vi "Configure Flow Rate.vi"(5 "Retry Attempts (0)":i32 min=0, 8 "error in":errorcluster, 10 "Flow Input (ml/min)":dbl, 11 "VISA resource name":refnum<visa-resource-name>) -> (0 "error out":errorcluster, 3 "VISA resource name out":refnum<visa-resource-name>)   [LabVIEW 2020, in "ChromTech Series III Pump.lvlib"]
doc: "Configures the flow rate using up to 5 digits. If the entered value exceeds the maximum allowable flow rate of the pump, the flow rate will be automatically set to the maximum allowable flow rate. The maximum allowable flow rate can be found using the Get Maximum Flow Rate VI and the current flow rate can be found using the Get Current Flow Rate VI or Get Current Conditions VI"
uses:
  ChromTech Series III Pump.lvlib
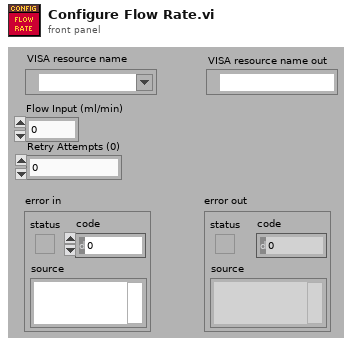
[diagram p1: front panel]
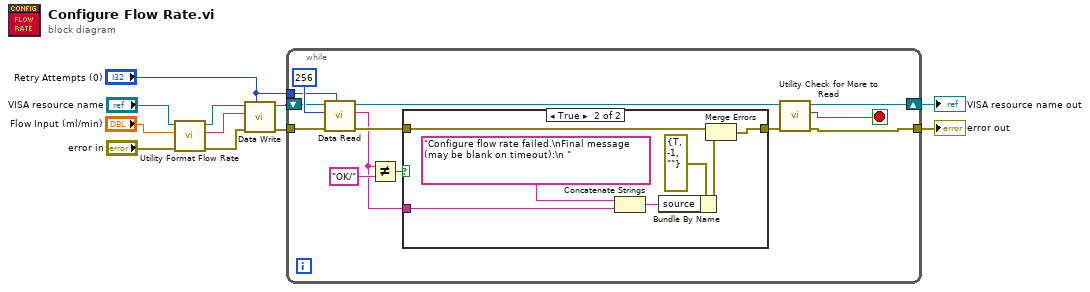
[diagram p0: block diagram]
diagram:
  n1 = call "Utility Format Flow Rate.vi"("error in (no error)"="error in", "Flow Rate"="Flow Input (ml/min)", "VISA resource name"="VISA resource name") -> ("error out"=w8:errorcluster, "Formatted Flow Rate"=w4:string, "VISA resource name out"=w3:refnum<visa-resource-name>)  [unwired: 6 in]
  n2 = call "Data Write.vi"("Retry Attempts (0)"="Retry Attempts (0)", "error in (no error)"=w8, "Command"=w4, "VISA Refnum in"=w3) -> ("error out"=w11:errorcluster, "VISA Refnum out"=w7:refnum<visa-resource-name>)  [unwired: 6 in]
  n3 = while {
    tunnel: "Retry Attempts (0)" -> [w16]
    shift-right: [w13] -> w10
    shift-left: w7 -> [w22]
    tunnel: w11 -> [w24]
    tunnel: [w15] -> w6
    stop <- w12 stop-if-true
    n4 = call "Data Read.vi"("Retry Attempts (0)"=w16, "error in (no error)"=w24, "Bytes to read"=256, "VISA Refnum in"=w22) -> ("error out"=w18:errorcluster, "read buffer"=w17:string, "VISA Refnum out"=w14:refnum<visa-resource-name>)  [unwired: 5 in]
    n5 = Not Equal?(x=w17, y="OK/") -> (x != y?=w20:bool)
    n6 = case shown="True" w20 {
      tunnel: [w25 w31] -> w19
      tunnel: w18 -> [w25 w30]
      tunnel: w17 -> [_ w26]
      frame False {
      }
      frame True {
        n7 = Concatenate Strings("Configure flow rate failed.\nFinal message (may be blank on timeout):\n ", w26) -> (w28:string)
        n8 = Bundle By Name(cluster=errorcluster {"status"=TRUE, "code"=-1, "source"=""} ("error out"), "source"=w28) -> (w29:errorcluster)
        n9 = Merge Errors(w30, w29) -> (w31:errorcluster)
      }
    }
    n10 = call "Utility Check for More to Read.vi"("error in (no error)"=w19, "VISA Refnum in"=w14) -> ("error out (unchanged)"=w15:errorcluster, "More to read?"=w12:bool, "VISA Refnum out"=w13:refnum<visa-resource-name>)  [unwired: 7 in]
  }
  "VISA resource name out" <- w10
  "error out" <- w6
